vi "ziExample-DIO.vi"() -> ()   [LabVIEW 2009]
doc: "Control a Zurich instrument device via the LabOne Labview API. \nRequirements: Zurich Instruments MFLI, HF2 or UHFLI \nThe example streams the auxiliary digital input.\n\n© Zurich Instruments AG, www.zhinst.com"
uses:
  <instrlib>/Zurich Instruments LabOne/Public/Data/ziGetEventDIOSample.vi
  <instrlib>/Zurich Instruments LabOne/Zurich Instruments LabOne.lvlib
panel:
  out "array of clusters":cluster{"Timestamp (ticks)":u64[][]}[](array[cluster])
  out "Error Out":errorcluster
  in  "Address":string="DEV"
  out "Selected Device":string
  out "Unexpected Node":string[](array[string])
  in  "stop":bool=TRUE
  out "Timestamps":u64[](graph)=[1435629509284, 1435629939412, 1435630369530, 1435630799650, 1435631229770, 1435631659890, 1435632090010, 1435632520130, 1435632950248, 1435633380368, 1435633810486, 1435634240606, 1435634670726, 1435635100846, 1435635530966, 1435635961084, 1435636391204, 1435636821322, 1435637251442, 1435637681562, 1435638111682, 1435638541810, 1435638971928, 1435639402048, 1435639832168, 1435640262288]
  out "Digital Data":u32[](graph)=[3, 3, 3, 3, 3, 3, 3, 3, 3, 3, 3, 3, 3, 3, 3, 3, 3, 3, 3, 3, 3, 3, 3, 3, 3, 3]
  # "ziExample-DIO.vi\nRequirements: HF2LI, UHFLI and MFLI\nsee block diagram for VI description"
  # "Tested Instruments:\n- MFLI\n- HF2LI\n- UHFLI"
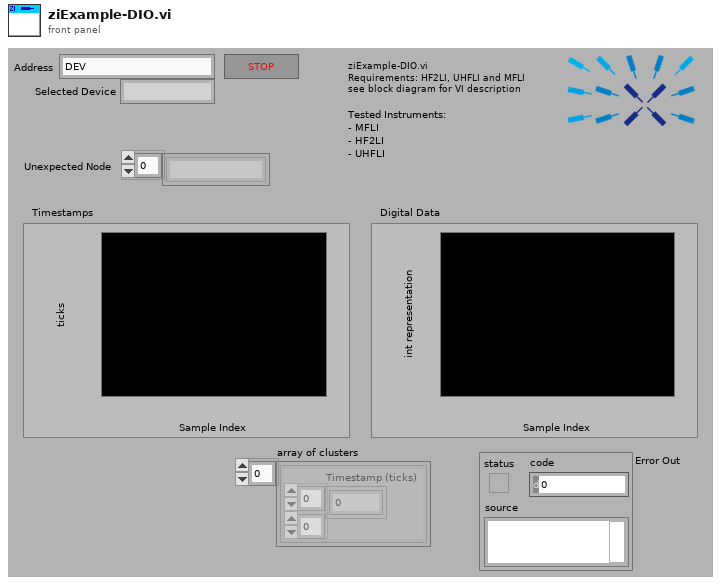
[diagram p1: front panel]
types:
  T1 = typedef "Zurich Instruments LabOne.lvlib/ziTypeHandle.ctl" = cluster{"handleValid":bool, "Conn":u64, "Path Prefix":string, "Handle":u64, "Connected":bool, "Clockbase(s)":dbl}
  T2 = cluster{"Timestamp (ticks)":u64[], "Value":u32[]}
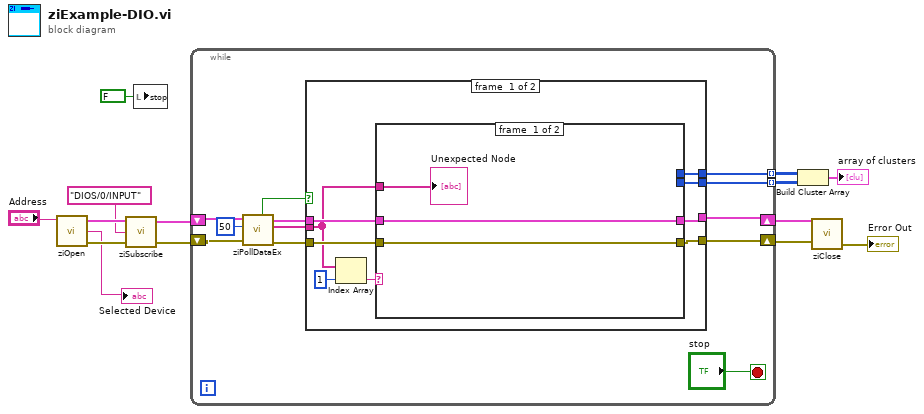
[diagram p0: block diagram]
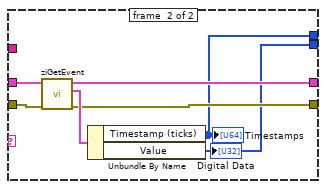
[diagram p2: hidden frame]
diagram:
  n1 = call <instrlib>:"ziOpen.vi"("Address"="Address") -> ("Error Out"=w11:errorcluster, "Selected Device"=→"Selected Device":string, "HandleOut"=w10:T1)  [unwired: 3 in]
  n2 = call <instrlib>:"ziSubscribe.vi"("error in"=w11, "Path ()"="DIOS/0/INPUT", "Handle In"=w10) -> ("error out"=w12:errorcluster, "Handle Out"=w9:T1)  [unwired: 1 in]
  n3 = local write "stop"(FALSE ("stop")) -> ()
  n4 = while {
    shift-right: [w18] -> w13
    shift-left: w9 -> [w25]
    shift-right: [w17] -> w14
    shift-left: w12 -> [w26]
    tunnel: [w16] -> w3 mode=indexing
    tunnel: [w15] -> w2 mode=indexing
    stop <- "stop" stop-if-true
    n5 = call <instrlib>:"ziPollDataEx.vi"("error in"=w26, "Timeout ms (50)"=50 ("TimeOut ms (50)"), "Handle In"=w25) -> ("error out"=w19:errorcluster, "PathArray"=w23:string[], "Handle Out"=w20:T1, "Timed Out"=w24:bool)  [unwired: 1 in, 4 out]
    n6 = case shown="False" w24 {
      tunnel: w23 -> [w29 _]
      tunnel: w20 -> [w35 w47]
      tunnel: w19 -> [w34 w46]
      tunnel: [w33 w47] -> w18
      tunnel: [w32 w46] -> w17
      tunnel: [w28 _] -> w16
      tunnel: [w27 _] -> w15
      frame #0 {
        n7 = Index Array(array=w29, index=1) -> (element=w30:string)
        n8 = case shown="\"DIOS\"" w30 {
          tunnel: w35 -> [w38 w45]
          tunnel: w34 -> [w37 w44]
          tunnel: [w38 w42] -> w33
          tunnel: [w37 w41] -> w32
          tunnel: w29 -> [w36 _]
          tunnel: [_ w40] -> w28
          tunnel: [_ w39] -> w27
          frame #0 {
            "Unexpected Node" <- w36
          }
          frame #1 {
            n9 = call-poly <instrlib>:"ziGetEvent.vi"("Error In"=w44, "Handle In"=w45) -> ("Error Out"=w41:errorcluster, "DIO Out"=w43:T2, "Handle Out"=w42:T1)  [unwired: 7 in]
            n10 = Unbundle By Name(w43) -> ("Timestamp (ticks)"=w40:u64[], "Value"=w39:u32[])
            "Digital Data" <- w39
            "Timestamps" <- w40
          }
        }
      }
      frame #1 {
      }
    }
  }
  n11 = Build Cluster Array(w3, w2) -> (→"array of clusters":cluster{"Timestamp (ticks)":u64[][]}[])
  n12 = call <instrlib>:"ziClose.vi"("Error In"=w14, "Handle In"=w13) -> ("Error Out"=→"Error Out":errorcluster)  [unwired: 2 in, 1 out]
